vi "mMc param - global.vi"() -> ()   [LabVIEW 2021]
panel:
  in  "deadband":dbl[](array[numeric]) format="%.2f"
  in  "PID":string[](array[string])
  in  "feedback":bool[](array[boolean])
  in  "done":bool
  in  "Jog Acc":dbl[](array[numeric]) format="%.2f"
  in  "Limit +":dbl[](array[numeric]) format="%.2f"
  in  "Limit -":dbl[](array[numeric]) format="%.2f"
  in  "Step Rezol":dbl[](array[numeric]) format="%.2f"
  in  "Enc Rezol":dbl[](array[numeric]) format="%.2f"
  in  "Positions":dbl[](array[numeric])=[0.0, 0.0, 0.0, 0.0, 0.0, 0.0, 0.0, 0.0, 0.0]
  in  "Motor ON":bool
  in  "Nr lines":i32
  in  "Active act":string
  in  "Active cont":string
  in  "Jog map":dbl[](array[numeric])=[0.0, 0.0003, 0.001, 0.003, 0.01, 0.03, 0.1, 0.3, 1.0] format="%.4f"
  in  "Jog":i32
  in  "Acceleration Max":dbl[](array[numeric]) format="%.2f"
  in  "Velocity Max":dbl[](array[numeric]) format="%.2f"
  in  "Last tick":u32=7251800
  in  "Destination":dbl[](array[numeric])=[-1.2819606487468604e-15, 0.0, 0.0, 0.0, 0.0, 0.0, 0.0, 0.0, 0.0] format="%.2f"
  in  "Acceleration":dbl[](array[numeric])=[8.0, 8.0, 8.0, 8.0, 8.0, 8.0, 8.0, 8.0, 8.0] format="%.2f"
  in  "Velocity":dbl[](array[numeric])=[2.0, 2.0, 2.0, 2.0, 2.0, 2.0, 2.0, 2.0, 2.0] format="%.2f"
  out "Position":i32[](array[numeric])
  # "Act"
  # "Cont"
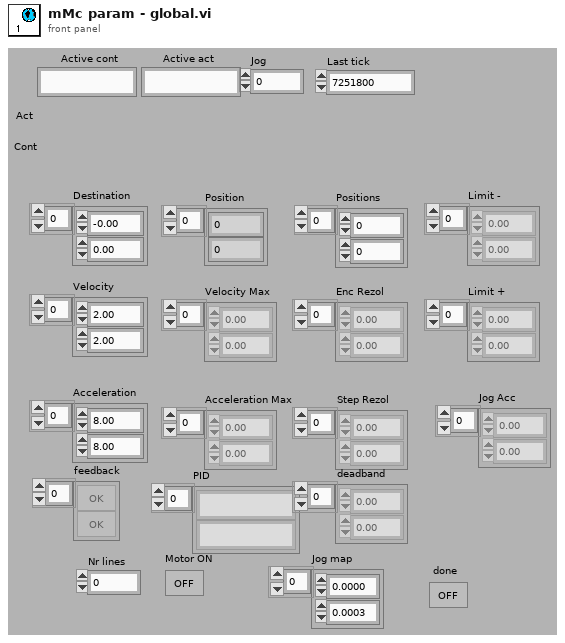
[diagram p1: front panel]
diagram:
